vi "oa_Order Magnitude dB Processing (1D array, N Channel Info).vi"(8 "dB on? (T)":bool=TRUE, 9 "x axis unit label":string, 10 "even angle channel info":T2[](array[typedef]) {"channel info"."pregain" format="%.2f"; "channel info"."weighting filter" items=["Linear", "A-weighting", "B-weighting", "C-weighting", "ITU-R 468-4", "Dolby", "CCITT", "C-message", "Wb", "Wc", "Wd", "We", "Wf", "Wh", "Wj", "Wk", "Wm", "AES17 20 kHz lowpass", "AES17 40 kHz lowpass", "AES17 20 kHz highpass", "AES17 40 kHz highpass"]; "channel info"."dB reference" format="%^.1e"; "channel info"."engineering units" items=["custom..."=0, "V"=1, "A"=21, "C"=30, "pC"=31, "s"=32, "-"=29, "Pa"=2, "N"=20, "g"=3, "m/s^2"=4, "m/s"=5, "m"=6, "mm/s"=12, "mm"=13, "micron/s"=14, "micron"=15, "in/s^2"=7, "in/s"=8, "in"=9, "mil/s"=10, "mil"=11, "rad/s^2"=16, "rad/s"=17, "rad"=18, "deg/s^2"=26, "deg/s"=27, "deg"=28, "RPM"=22, "cycle/s^2"=23, "Hz"=24, "cycle"=25, "strain"=19]; "channel info"."sensor sensitivity" format="%#_5f"}, 11 "magnitudes":T6(array[cluster]) {"magnitude" format="%.2f"; "time/rev/rpm" format="%.2f"}) -> (1 "unit labels":T1(array[cluster]), 3 "magnitudes dB":T6(array[cluster]) {"magnitude" format="%.2f"; "time/rev/rpm" format="%.2f"})   [LabVIEW 2017, in "SoundVib_Resampling.lvlib"]
uses:
  <vilib>/addons/Sound and Vibration/Order Analysis/Resample Order Tracking/SoundVib_Resampling.lvlib
  <vilib>/addons/_NISVFA/_Shared subVIs/Controls/svc_Resampled Channel Info.ctl
  <vilib>/addons/_NISVFA/_Shared subVIs/Controls/svc_Channel Info.ctl
  <vilib>/addons/_NISVFA/_Shared subVIs/Controls/svc_Engineering Units Text Ring.ctl
  <vilib>/addons/_NISVFA/_Shared subVIs/Controls/svc_Weighting Filter Text Ring.ctl
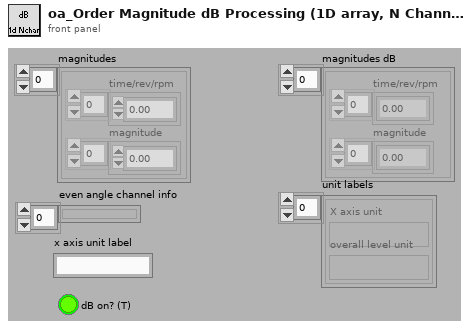
[diagram p1: front panel]
types:
  T1 = cluster{"X axis unit":string, "overall level unit":string}[]
  T2 = typedef "svc_Resampled Channel Info.ctl" = cluster{"channel name":string, "description":string, " channel info":T3}
  T3 = typedef "svc_Channel Info.ctl" = cluster{"sensor sensitivity":dbl, "engineering units":T4, "dB reference":dbl, "custom label":string, "weighting filter":T5, "pregain":dbl}
  T4 = typedef "svc_Engineering Units Text Ring.ctl" = u16
  T5 = typedef "svc_Weighting Filter Text Ring.ctl" = u16
  T6 = cluster{"time/rev/rpm":dbl[], "magnitude":dbl[]}[]
  T7 = cluster{"x axis unit label":string, "unit label":string}
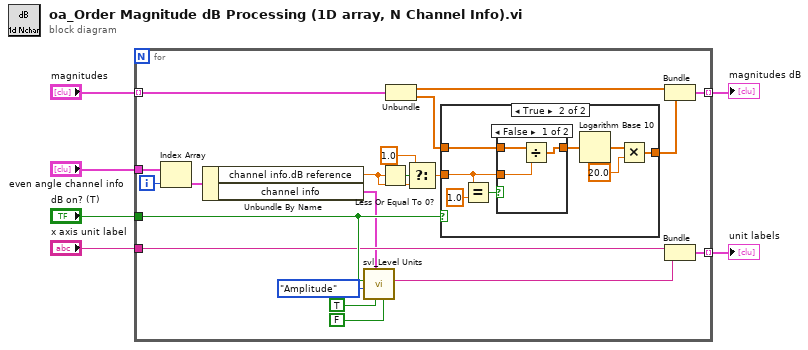
[diagram p0: block diagram]
diagram:
  n1 = for {
    tunnel: "magnitudes" -> [w26] mode=indexing
    tunnel: [w24] -> w5 mode=indexing
    tunnel: "dB on? (T)" -> [w17]
    tunnel: "even angle channel info" -> [w9]
    tunnel: "x axis unit label" -> [w15]
    tunnel: [w12] -> w1 mode=indexing
    i -> [w7]
    n2 = Index Array(array=w9, index=w7) -> (element=w8:T2)
    n3 = Unbundle By Name(w8) -> ("channel info.dB reference"=w21:dbl, "channel info"=w14:T3)
    n4 = call <vilib>:"svl_Level Units.vi"("include weighting if dB On FALSE"=FALSE, "rms level (T)"=TRUE, "channel info"=w14, "view mode"=enum16{"Power", "Amplitude"}."Amplitude", "dB On (T)"=w17) -> ("unit label"=w13:string)  [unwired: 4 in, 2 out]
    n5 = Less Or Equal To 0?(x=w21) -> (x <= 0?=w19:bool)
    n6 = Unbundle(w26) -> ("time/rev/rpm"=w25:dbl[], "magnitude"=w23:dbl[])
    n7 = Select(t=1.0, s=w19, f=w21) -> (s? t:f=w18:dbl)
    n8 = case shown="True" w17 {
      tunnel: w23 -> [w27 w30]
      tunnel: [w27 w33] -> w22
      tunnel: w18 -> [_ w28]
      frame False {
      }
      frame True {
        n9 = Equal?(x=w28, y=1.0) -> (x = y?=w31:bool)
        n10 = case shown="False" w31 {
          tunnel: w30 -> [w38 w39]
          tunnel: [w36 w39] -> w29
          tunnel: w28 -> [w37 _]
          frame False {
            n11 = Divide(x=w38, y=w37) -> (x/y=w36:dbl[])
          }
          frame True {
          }
        }
        n12 = Logarithm Base 10(1:w29) -> (0:w35:dbl[])
        n13 = Multiply(x=w35, y=20.0) -> (x*y=w33:dbl[])
      }
    }
    n14 = Bundle("time/rev/rpm"=w25, "magnitude"=w22) -> (w24:cluster{"time/rev/rpm":dbl[], "magnitude":dbl[]})  [unwired: 1 in]
    n15 = Bundle("x axis unit label"=w15, "unit label"=w13) -> (w12:T7)  [unwired: 1 in]
  }
  "magnitudes dB" <- w5
  "unit labels" <- w1
